vi "Fit_felix.3.vi"() -> ()   [LabVIEW 2016]
uses:
  <vilib>/gmath/NumericalOptimization/Nonlinear Curve Fit LM bound.vi
  <vilib>/gmath/NI_Gmath.lvlib
panel:
  out "error out":errorcluster
  out "Baseline d x + e":dbl[][](array[numeric]) format="%.3f"
  out "a4 exp(-0.5((x-b4)/c)^2)":dbl[][](array[numeric]) format="%.3f"
  out "a3 exp(-0.5((x-b3)/c)^2)":dbl[][](array[numeric]) format="%.3f"
  out "a2 exp(-0.5((x-b2)/c)^2)":dbl[][](array[numeric]) format="%.3f"
  out "a1 exp(-0.5((x-b1)/c)^2)":dbl[][](array[numeric]) format="%.3f"
  out "Residue":dbl[](array[numeric]) format="%#_3e"
  out "Last Spectrum":cluster{"Array":dbl[], "Array":dbl[]}[](graph)
  in  "Fit Termination":cluster{"max iteration":i32, "tolerance":dbl}={"max iteration"=200, "tolerance"=1e-08}
  in  "Initial":dbl[](array[numeric])=[0.2, 55.3, 0.9, 0.54, 57.9, 0.9, 0.6, 60.6, 0.9, 0.46, 62.207, 0.9, -0.024, 0.7]
  out "Last Spectrum":dbl[][](array[numeric]) caption="Array"
  in  "Path":path
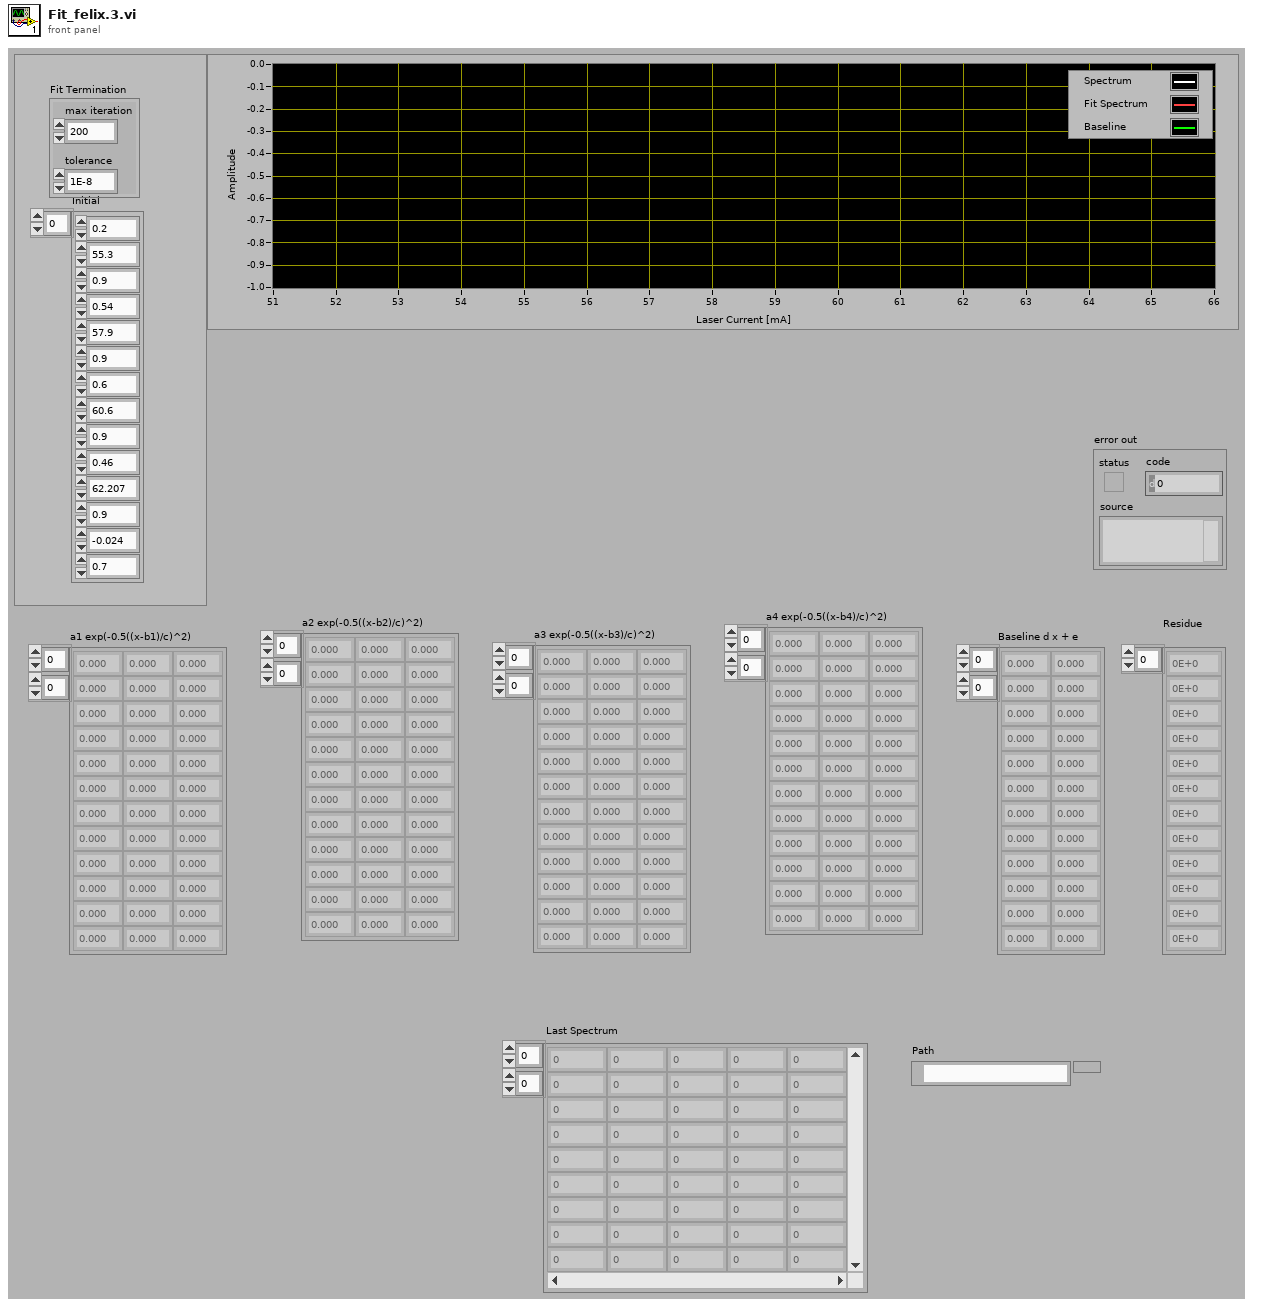
[diagram p1: front panel]
types:
  T1 = cluster{"Last spectrum loaded":dbl[], "Last spectrum loaded":dbl[]}
  T2 = cluster{"Last spectrum loaded":dbl[], "best nonlinear fit":dbl[]}
  T3 = cluster{"Last spectrum loaded":dbl[], "best nonlinear fit":dbl[]}[]
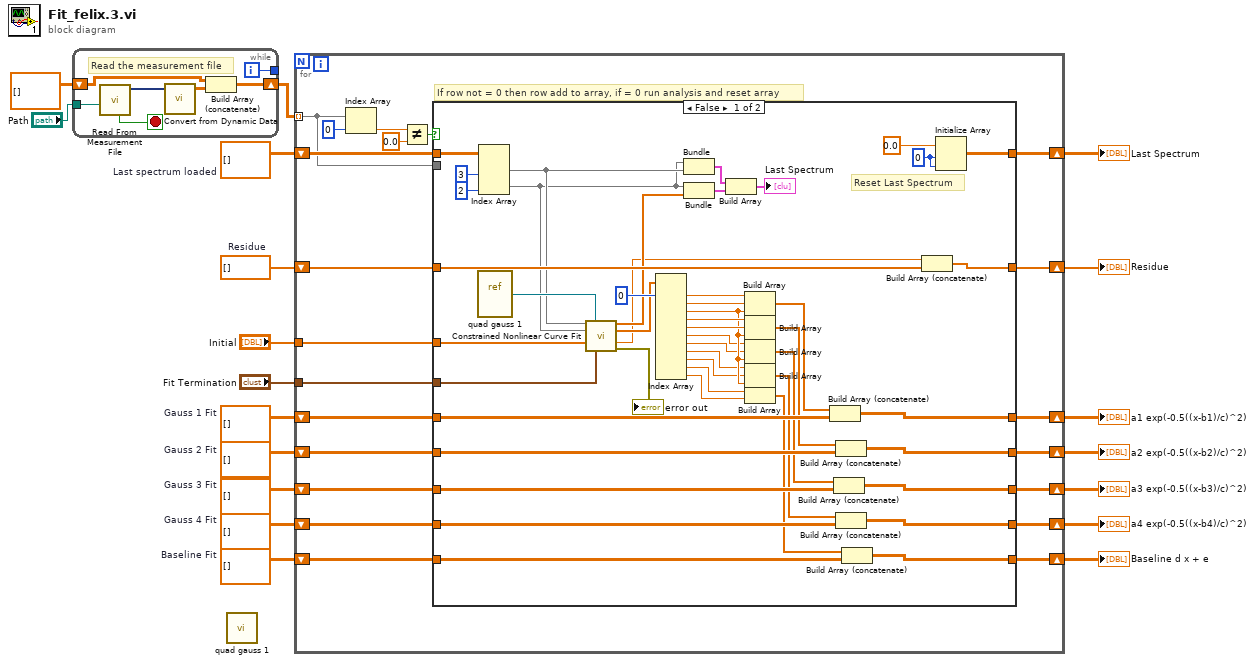
[diagram p0: block diagram]
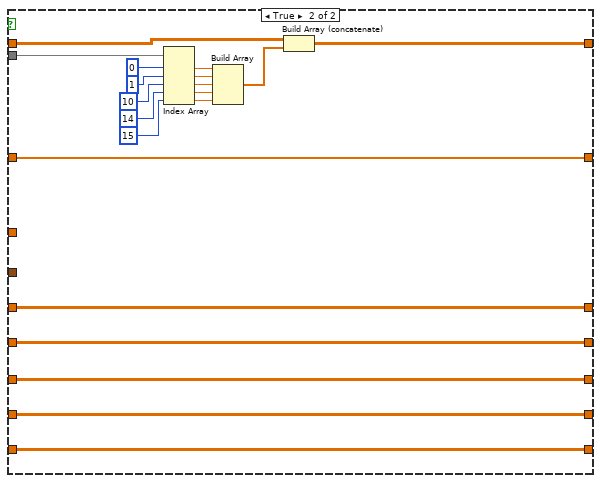
[diagram p2: hidden frame]
diagram:
  w9 = dbl[][] []  # Baseline Fit
  w10 = dbl[][] []  # Gauss 4 Fit
  w11 = dbl[][] []  # Gauss 3 Fit
  (unwired) dbl[][] []  # Gauss 2 Fit
  w13 = dbl[][] []  # Gauss 1 Fit
  w14 = dbl[] []  # Residue
  w15 = dbl[][] []  # Last spectrum loaded
  n1 = while {
    shift-right: [w25] -> w19
    shift-left: dbl[][] [] -> [w23]
    tunnel: "Path" -> [w22]
    tunnel: [w20] -> _
    i -> [w20]
    stop <- w24 stop-if-true
    # "Read the measurement file"
    n2 = call "Read From Measurement File"("Filename"=w22) -> ("Signals"=w21:dynamicdata, "EOF?"=w24:bool)  [unwired: 5 in, 4 out]
    n3 = call "Convert from Dynamic Data"("Dynamic Data Type"=w21) -> ("Array"=w26:dbl[][])  [unwired: 3 out]
    n4 = Build Array (concatenate)(w23, w26) -> (w25:dbl[][])
  }
  n5 = call "quad gauss 1.vi"() -> ()  [unwired: 4 in, 3 out]
  n6 = for {
    tunnel: w19 -> [w41] mode=indexing
    shift-right: [w42] -> w16
    shift-left: w15 -> [w43]
    shift-right: [w29] -> w3
    shift-left: w14 -> [w40]
    shift-right: [w38] -> w6
    shift-left: w13 -> [w39]
    shift-right: [w37] -> w4
    shift-left: dbl[][] [] ("element") -> [w36]
    shift-right: [w34] -> w8
    shift-left: w11 -> [w35]
    shift-right: [w33] -> w7
    shift-left: w10 -> [w32]
    shift-right: [w30] -> w5
    shift-left: w9 -> [w31]
    tunnel: "Initial" -> [w28]
    tunnel: "Fit Termination" -> [w27]
    # "If row not = 0 then row add to array, if = 0 run analysis and reset array"
    n7 = Index Array(array=w41, index=0) -> (element=w45:dbl)
    n8 = Not Equal?(x=w45, y=0.0) -> (x != y?=w46:bool)
    n9 = case shown="False" w46 {
      tunnel: w41 -> [_ w112]
      tunnel: w43 -> [w69 w114]
      tunnel: [w93 w102] -> w42
      tunnel: w40 -> [w91 w95]
      tunnel: [w71 w95] -> w29
      tunnel: w39 -> [w87 w100]
      tunnel: [w85 w100] -> w38
      tunnel: w36 -> [w83 w99]
      tunnel: [w70 w99] -> w37
      tunnel: w35 -> [w82 w98]
      tunnel: [w80 w98] -> w34
      tunnel: w32 -> [w77 w97]
      tunnel: [w79 w97] -> w33
      tunnel: w31 -> [w75 w96]
      tunnel: [w74 w96] -> w30
      tunnel: w28 -> [w49 _]
      tunnel: w27 -> [w48 _]
      frame False {
        w66 = 0 ("dimension size")
        # "Reset Last Spectrum"
        n10 = vi-ref "quad gauss 1.vi"() -> (w63:refnum<vi>)
        n11 = Index Array(array=w69, index (col) #1=3 ("index (col)"), index (col) #2=2 ("disabled index (col)")) -> (element #1=w62:dbl[], element #2=w61:dbl[])  [unwired: 2 in]
        n12 = call-poly <vilib>:"Constrained Nonlinear Curve Fit.vi"("Y"=w62, "f(x,a)"=w63, "X"=w61, "initial parameters"=w49, "termination"=w48) -> ("best nonlinear fit"=w58:dbl[], "best fit parameters"=w59:dbl[], "residue"=w57:dbl, "error out"=→"error out":errorcluster)  [unwired: 5 in, 2 out]
        n13 = Index Array(array=w59, index #1=0 ("index")) -> (element #1=w73:dbl, element #2=w72:dbl, element #3=w56:dbl, element #4=w65:dbl, element #5=w64:dbl, element #6=w55:dbl, element #7=w54:dbl, element #8=w53:dbl, element #9=w52:dbl, element #10=w51:dbl, element #11=w50:dbl)  [unwired: 10 in]
        n14 = Bundle("Last spectrum loaded"=w61, "Last spectrum loaded"=w62) -> (w90:T1)  [unwired: 1 in]
        n15 = Bundle("Last spectrum loaded"=w61, "best nonlinear fit"=w58) -> (w89:T2)  [unwired: 1 in]
        n16 = Build Array(w90, w89) -> (→"Last Spectrum":T3)
        n17 = Build Array(w73, w72, w56) -> (w86:dbl[])
        n18 = Build Array(w65, w64, w56) -> (w84:dbl[])
        n19 = Build Array(w55, w54, w56) -> (w81:dbl[])
        n20 = Build Array(w53, w52, w56) -> (w78:dbl[])
        n21 = Build Array(w51, w50) -> (w76:dbl[])
        n22 = Build Array (concatenate)(w86, w87) -> (w85:dbl[][])
        n23 = Build Array (concatenate)(w81, w82) -> (w80:dbl[][])
        n24 = Build Array (concatenate)(w84, w83) -> (w70:dbl[][])
        n25 = Build Array (concatenate)(w78, w77) -> (w79:dbl[][])
        n26 = Build Array (concatenate)(w76, w75) -> (w74:dbl[][])
        n27 = Build Array (concatenate)(w57, w91) -> (w71:dbl[])
        n28 = Initialize Array(0.0 ("element"), w66, w66) -> (w93:dbl[][])
      }
      frame True {
        n29 = Index Array(array=w112, index #1=0 ("index"), index #2=1 ("index"), index #3=10 ("index"), index #4=14 ("index"), index #5=15 ("index")) -> (element #1=w107:dbl, element #2=w106:dbl, element #3=w105:dbl, element #4=w104:dbl, element #5=w103:dbl)
        n30 = Build Array(w107, w106, w105, w104, w103) -> (w101:dbl[])
        n31 = Build Array (concatenate)(w114, w101) -> (w102:dbl[][])
      }
    }
  }
  "Last Spectrum" <- w16
  "Residue" <- w3
  "a1 exp(-0.5((x-b1)/c)^2)" <- w6
  "a2 exp(-0.5((x-b2)/c)^2)" <- w4
  "a3 exp(-0.5((x-b3)/c)^2)" <- w8
  "a4 exp(-0.5((x-b4)/c)^2)" <- w7
  "Baseline d x + e" <- w5
